vi "Loop Timer.vi"(8 "error in (no error)":errorcluster) -> (0 "error out":errorcluster, 3 "Loop Time":dbl)   [LabVIEW 2013]
doc: "Simple functional global variable, outputs time of one loop iteration."
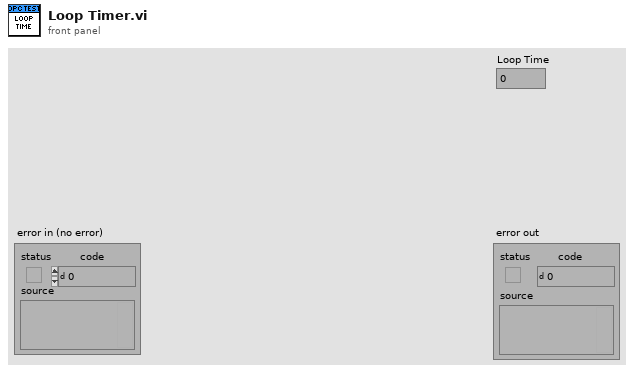
[diagram p1: front panel]
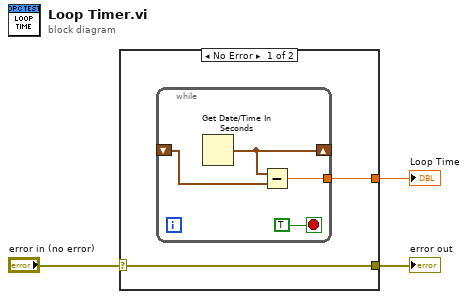
[diagram p0: block diagram]
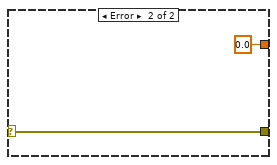
[diagram p2: hidden frame]
diagram:
  n1 = case shown="No Error" "error in (no error)" {
    selector: "error in (no error)" -> [w4 w11]
    tunnel: [w4 w11] -> w2
    tunnel: [w5 0.0] -> w1
    frame No Error {
      n2 = while {
        shift-right: [w9] -> _
        shift-left: _ -> [w8]
        tunnel: [w6] -> w5
        stop <- TRUE stop-if-true
        n3 = Get Date/Time In Seconds() -> (seconds since 1Jan1904=w9:timestamp)
        n4 = Subtract(x=w9, y=w8) -> (x-y=w6:dbl)
      }
    }
    frame Error {
    }
  }
  "error out" <- w2
  "Loop Time" <- w1
